vi "Trav_move_above_height.vi"(4 "Currently on Point":i32=11, 6 "Row Number":i32=11, 7 "Extra Command String":string, 8 "Simulate/Run":T1, 9 "Backlash Compensation?":bool=TRUE, 10 "New Position":dbl[](array[numeric])=[0.0, 0.0, 0.0] format="%.2f", 11 "Mode":T2) -> (0 "Error String":string, 3 "Trav Position achieved":dbl[](array[numeric]) format="%.2f")   [LabVIEW 2012]
uses:
  Trav_mode.ctl
  Controls/User_Specific_mode.ctl
  Controls/Tunnel_Coordinates.ctl
  Globals/Trav_pos_global.vi
  Globals/Extra_Commands_Global.vi
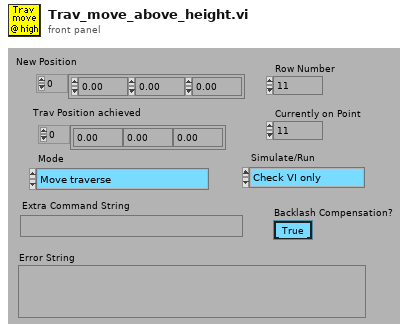
[diagram p1: front panel]
types:
  T1 = typedef "User_Specific_mode.ctl" = enum16{"Check VI only", "Run VI"}
  T2 = typedef "Trav_mode.ctl" = enum16{"Move traverse", "Read traverse position", "Teach Position"}
  T3 = typedef "Tunnel_Coordinates.ctl" = enum16{"Work in Tunnel Coordinates", "Work in Model Coordinates"}
  T4 = enum16{"To Traverse Coordinates", "To User Coordinates"}
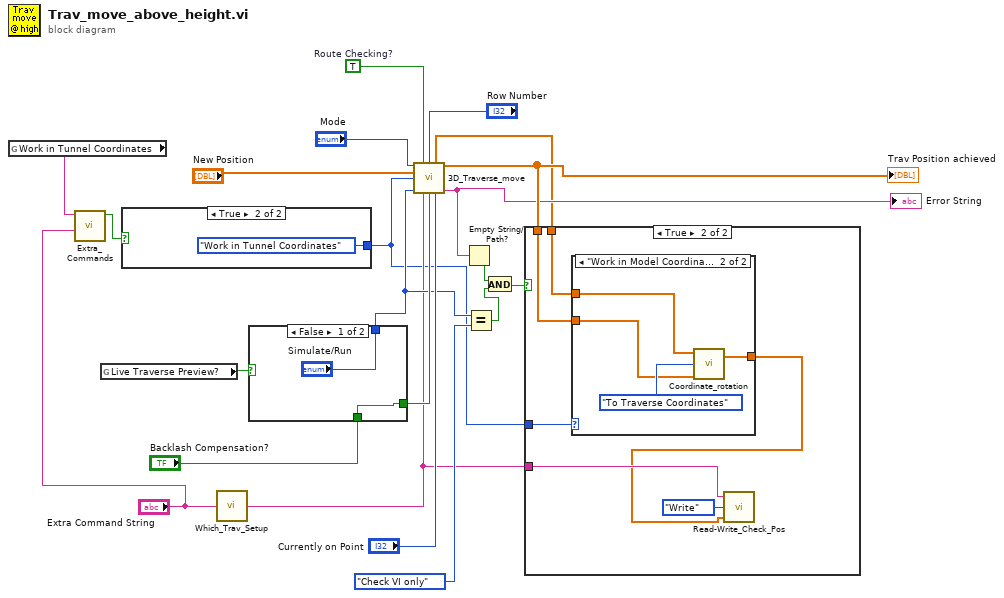
[diagram p0: block diagram]
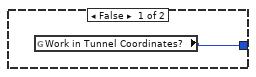
[diagram p2: hidden frame]
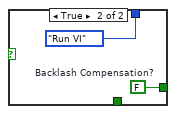
[diagram p5: hidden frame]
diagram:
  w13 = TRUE  # Route Checking?
  n1 = global read "Extra_Commands_Global.vi" "Work in Tunnel Coordinates"() -> (w4:string)
  n2 = call "Extra_Commands.vi"("String to Search"="Extra Command String", "Command"=w4) -> ("Command Found"=w2:bool)  [unwired: 1 in, 4 out]
  n3 = global read "Trav_pos_global.vi" "Live Traverse Preview?"() -> (w15:bool)
  n4 = case shown="True" w2 {
    tunnel: [w22 Tunnel_Coordinates."Work in Tunnel Coordinates" ("Work in Tunnel Coordinates?")] -> w1
    frame False {
      n5 = global read "Trav_pos_global.vi" "Work in Tunnel Coordinates?"() -> (w22:T3)
    }
    frame True {
    }
  }
  n6 = call "Which_Trav_Setup.vi"("Extra Command String"="Extra Command String") -> ("Traverse Setup"=w7:string)
  n7 = case shown="False" w15 {
    tunnel: ["Simulate/Run" User_Specific_mode."Run VI" ("Simulate/Run")] -> w11
    tunnel: [w24 w26] -> w14
    tunnel: "Backlash Compensation?" -> [w24 _]
    frame False {
    }
    frame True {
      w26 = FALSE  # Backlash Compensation?
    }
  }
  n8 = call "3D_Traverse_move.vi"("Mode"="Mode", "Route Checking?"=w13, "Row Number"="Row Number", "Position"="New Position", "Work in Tunnel Coordinates"=w1, "Simulate/Run"=w11, "Traverse name"=w7, "Backlash Compensation?"=w14, "Currently on Point"="Currently on Point") -> ("Model  Roll        Pitch       Yaw (deg)"=w5:dbl[], "Trav Position achieved"=w20:dbl[], "Error String"=w19:string)  [unwired: 4 out]
  "Trav Position achieved" <- w20
  "Error String" <- w19
  n9 = Empty String/Path?(string/path=w19) -> (empty?=w10:bool)
  n10 = Equal?(x=w11, y=User_Specific_mode."Check VI only" ("Simulate/Run")) -> (x = y?=w9:bool)
  n11 = And(x=w10, y=w9) -> (x .and. y?=w8:bool)
  n12 = case shown="True" w8 {
    tunnel: w5 -> [_ w33]
    tunnel: w20 -> [_ w32]
    tunnel: w1 -> [_ w31]
    tunnel: w7 -> [_ w29]
    frame False {
    }
    frame True {
      n13 = case shown="\"Work in Model Coordinates\"" w31 {
        tunnel: w32 -> [w34 w37]
        tunnel: [w34 w36] -> w28
        tunnel: w33 -> [_ w35]
        frame "Work in Tunnel Coordinates" {
        }
        frame "Work in Model Coordinates" {
          n14 = call "Coordinate_rotation.vi"("Model       Roll      Pitch       Yaw (deg)"=w35, "Input Position"=w37, "Mode"=T4."To Traverse Coordinates") -> ("Output Position"=w36:dbl[])  [unwired: 2 in, 1 out]
        }
      }
      n15 = call "Read-Write_Check_Pos.vi"("Position input"=w28, "Mode"=enum16{"Read", "Write"}."Write", "Traverse Name"=w29) -> ()  [unwired: 1 out]
    }
  }
